vi "EditOptions.vi"(8 "error in":errorcluster, 11 "channel in":refnum<class "Channel.lvclass">) -> (0 "error out":errorcluster, 1 "edit options":T1, 2 "subnodes class":T2, 3 "channel out":refnum<class "Channel.lvclass">)   [LabVIEW 2013, in "Channel.lvclass"]
doc: "This VI Contains the options for the Menu that will be displayed when doing right click on an item\nThe subnodes class configures which nodes can be added to this nodes\nAnd the edit options determine which options are available for the node.\n\nThis configuration is stored in this VI in case some dynamic configuration is required for the menu options or subnodes.\n\nAll VIs must overide this method"
uses:
  Channel.lvclass
  CEF_TreeControl/Node/SubNodeCluster.ctl
  CEF_TreeControl/Node/NodeMenuOptions.ctl
  CEF_TreeControl/Node/NISE_CEF_Node.lvclass
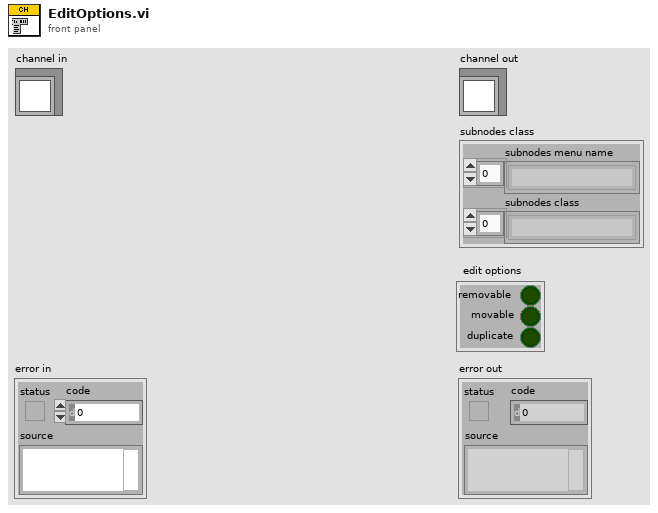
[diagram p1: front panel]
types:
  T1 = typedef "NISE_CEF_Node.lvclass/NodeMenuOptions.ctl" = cluster{"removable":bool, "movable":bool, "duplicate":bool}
  T2 = typedef "NISE_CEF_Node.lvclass/SubNodeCluster.ctl" = cluster{"subnodes menu name":string[], "subnodes class":string[]}
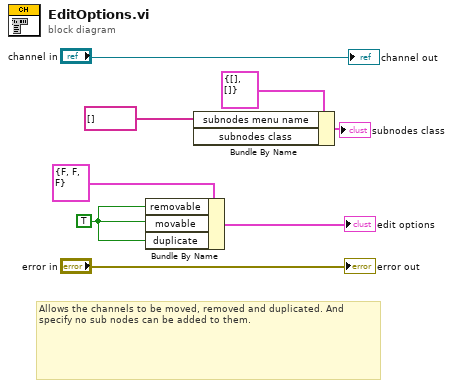
[diagram p0: block diagram]
diagram:
  w5 = TRUE ("movable")
  w3 = string[] [] ("subnodes class")
  # "Allows the channels to be moved, removed and duplicated. And specify no sub nodes can be added to them."
  n1 = Bundle By Name(cluster=T1 {"removable"=FALSE, "movable"=FALSE, "duplicate"=FALSE} ("edit options 2"), "removable"=w5, "movable"=w5, "duplicate"=w5) -> (→"edit options":T1)
  n2 = Bundle By Name(cluster=T2 {"subnodes menu name"=[], "subnodes class"=[]} ("subnodes class"), "subnodes menu name"=w3, "subnodes class"=w3) -> (→"subnodes class":T2)
  "error out" <- "error in"
  "channel out" <- "channel in"
